vi "Configure Modulation (Custom Advanced).vi"(0 "VISA resource name":refnum<visa-resource-name>, 5 "ASK Depth (100 %)":dbl=100.0, 11 "error in (no error)":errorcluster) -> (4 "VISA resource name out":refnum<visa-resource-name>, 15 "error out":errorcluster)   [LabVIEW 2014, in "Agilent PSG MXG Series.lvlib"]
doc: "Configures the depth for the amplitude shift keying (ASK) modulation.\n\n<B>Notes:</B>\n(1) This VI is valid only in N5172B, N5182B."
uses:
  Agilent PSG MXG Series.lvlib
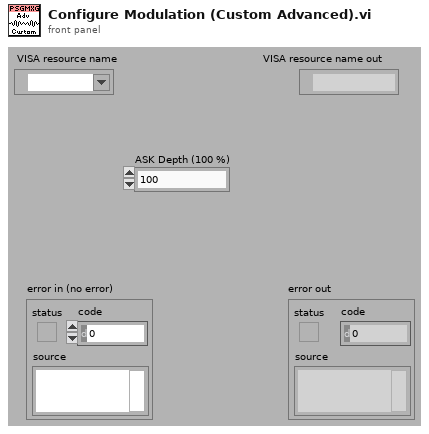
[diagram p1: front panel]
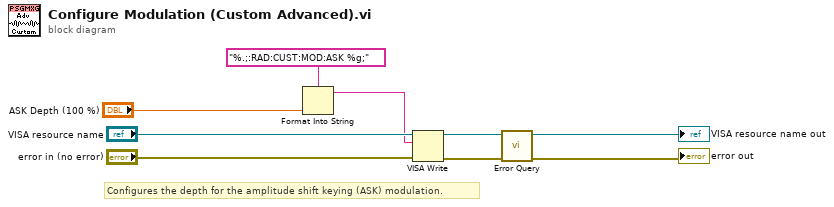
[diagram p0: block diagram]
diagram:
  # "Configures the depth for the amplitude shift keying (ASK) modulation."
  n1 = Format Into String(format string="%.;:RAD:CUST:MOD:ASK %g;", "ASK Depth (100 %)") -> (resulting string=w1:string)  [unwired: 2 in, 1 out]
  n2 = VISA Write(VISA resource name="VISA resource name", write buffer=w1, error in (no error)="error in (no error)") -> (VISA resource name out=w9:refnum<visa-resource-name>, error out=w8:errorcluster)  [unwired: 1 out]
  n3 = call "Error Query.vi"("error in (no error)"=w8, "VISA resource name"=w9) -> ("error out"=→"error out":errorcluster, "VISA resource name out"=→"VISA resource name out":refnum<visa-resource-name>)  [unwired: 8 out]
